vi "Windows_SystemTime_to_String.vi"(1 "time format string (%c)":string="%c", 2 "UTC Date and Time in":T1={"Year"=0, "Month"=1, "DayOfWeek"=0, "Day"=0, "Hour"=0, "Minute"=0, "Seconds"=0, "Milliseconds"=0} {"DayOfWeek" items=["Sunday", "Monday", "Tuesday", "Wednesday", "Thursday", "Friday", "Saturday"]; "Month" items=["", "January", "February", "March", "April", "May", "June", "July", "August", "September", "October", "November", "December"]}) -> (0 "UTC Date and Time out (string)":string)   [LabVIEW 2012]
doc: "This VI takes in a Windows SYSTEMTIME structure and displays the date and time in seconds since 12:00 a.m., January 1, 1904, Universal time, in a format you specify.\n\nThe SYSTEMTIME structure consists of:\n<B>Year</B>\nSpecifies the current year.\n<B>Month</B>\nSpecifies the current month; January = 1, February = 2, and so on.\n<B>DayOfWeek</B>\nSpecifies the current day of the week; Sunday = 0, Monday = 1, and so on.\n<B>Day</B>\nSpecifies the current day of the month.\n<B>Hour</B>\nSpecifies the current hour.\n<B>Minute</B>\nSpecifies the current minute.\n<B>Second</B>\nSpecifies the current second.\n<B>Milliseconds</B>\nSpecifies the current millisecond.\n\nThe <B>time format string</B> can contain any combination of the following codes: %H (hour, 24-hour clock), %I (hour, 12-hour clock), %M (minute), %S (second), %p (a.m./p.m. flag), %d (day of month), %m (month number), %y (year within century), %Y (year including century), %a (abbreviated weekday name), %x (locale-specific date), %X (locale-specific time), %c (locale-specific date/time), %<digit>u (fractional seconds with <digit> precision)."
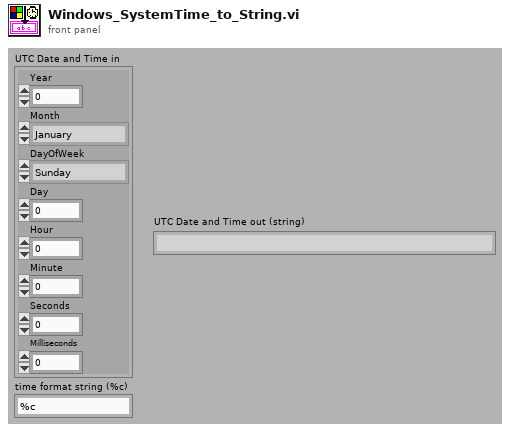
[diagram p1: front panel]
types:
  T1 = cluster{"Year":u16, "Month":u16, "DayOfWeek":u16, "Day":u16, "Hour":u16, "Minute":u16, "Seconds":u16, "Milliseconds":u16}
  T2 = cluster{"Seconds":i32, "Minute":i32, "Hour":i32, "Day":i32, "Month":i32, "Year":i32, "DayOfWeek":i32, i32, i32}
  T3 = cluster{"Year":i32, "Month":i32, "DayOfWeek":i32, "Day":i32, "Hour":i32, "Minute":i32, "Seconds":i32, "Milliseconds":i32}
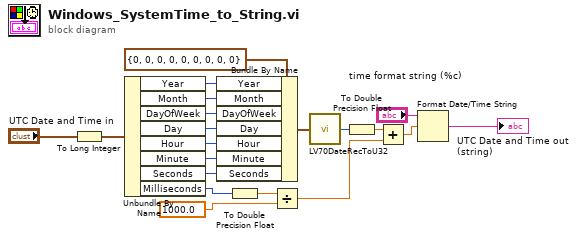
[diagram p0: block diagram]
diagram:
  n1 = To Long Integer(number="UTC Date and Time in") -> (32bit integer=w19:T3)
  n2 = Unbundle By Name(w19) -> ("Year"=w17:i32, "Month"=w11:i32, "DayOfWeek"=w13:i32, "Day"=w12:i32, "Hour"=w14:i32, "Minute"=w15:i32, "Seconds"=w16:i32, "Milliseconds"=w9:i32)
  n3 = Bundle By Name(cluster=T2 {"Seconds"=0, "Minute"=0, "Hour"=0, "Day"=0, "Month"=0, "Year"=0, "DayOfWeek"=0, 0, 0} ("output cluster"), "Year"=w17, "Month"=w11, "DayOfWeek"=w13, "Day"=w12, "Hour"=w14, "Minute"=w15, "Seconds"=w16) -> (w10:T2)
  n4 = To Double Precision Float(number=w9) -> (double precision float=w2:dbl)
  n5 = Divide(x=w2, y=1000.0) -> (x/y=w6:dbl)
  n6 = call <vilib>:"LV70DateRecToU32.vi"("date time rec"=w10) -> ("Time"=w7:u32)
  n7 = To Double Precision Float(number=w7) -> (double precision float=w1:dbl)
  n8 = Add(x=w1, y=w6) -> (x+y=w5:dbl)
  n9 = Format Date/Time String(time format string (%c)="time format string (%c)", seconds (now)=w5) -> (date/time string=→"UTC Date and Time out (string)":string)  [unwired: 1 in]
